vi "prep state ui.vi"(4 "Output Tag":refnum<vi>, 6 "Input Tag":refnum<vi>, 8 "error in":errorcluster, 10 "engine configuration in":refnum<class "engine configuration.lvclass">, 11 "user tag bus module configuration in":refnum<class "TEST CONFIGURATION.lvclass">) -> (0 "error out":errorcluster, 2 "engine configuration out":refnum<class "engine configuration.lvclass">)   [LabVIEW 2013, in "configuration tests.lvlib" / "TEST EDITOR.lvclass"]
uses:
  TEST EDITOR.lvclass
  module/configuration/TEST CONFIGURATION.lvclass
  <vilib>/NI/Module Execution Interface/Engine Configuration/engine configuration.lvclass
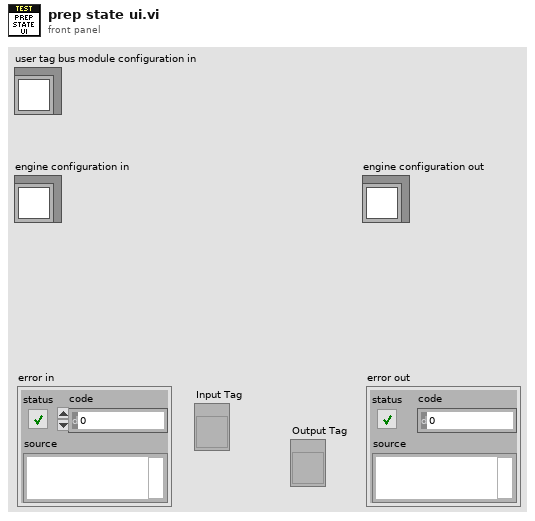
[diagram p1: front panel]
types:
  T1 = typedef "user tag bus module configuration.lvclass/state module configuration.ctl" = cluster{"fixed input":refnum<class "TBM channel.lvclass">, "fixed output":refnum<class "TBM channel.lvclass">, "initial state":u8}
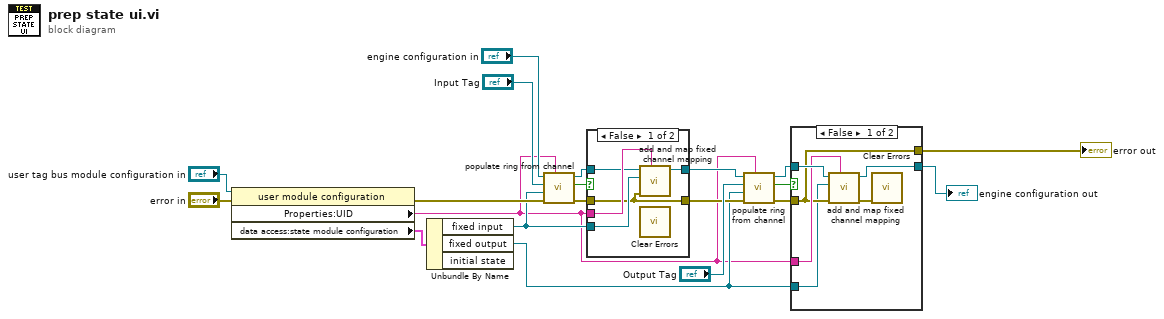
[diagram p0: block diagram]
diagram:
  n1 = property class="user module configuration"(reference="user tag bus module configuration in", error in="error in") -> (error out=w16:errorcluster, "Properties:UID"=w6:string, "data access:state module configuration"=w17:T1)  [unwired: 1 out]
  n2 = Unbundle By Name(w17) -> ("fixed input"=w10:refnum<class "TBM channel.lvclass">, "fixed output"=w7:refnum<class "TBM channel.lvclass">)  [unwired: 1 out]
  n3 = call "populate ring from channel.vi"("instance id"=w6, "error in"=w16, "channel"=w10, "ring"="Input Tag", "engine configuration in"="engine configuration in") -> ("error out"=w9:errorcluster, "mapped"=w13:bool, "engine configuration out"=w11:refnum<class "engine configuration.lvclass">)  [unwired: 4 in]
  n4 = case shown="False" w13 {
    tunnel: [w25 w27] -> w12
    tunnel: w11 -> [w22 w27]
    tunnel: w9 -> [w21 w26]
    tunnel: w10 -> [w24 _]
    tunnel: w6 -> [w23 _]
    tunnel: [w21 w26] -> w8
    frame False {
      n5 = call <vilib>:"add and map fixed channel mapping.vi"("module instance"=w23, "error in"=w21, "fixed channel"=w24, "engine configuration in"=w22) -> ("engine configuration out"=w25:refnum<class "engine configuration.lvclass">)  [unwired: 6 in, 1 out]
      n6 = call <vilib>:"Clear Errors.vi"() -> ()  [unwired: 7 in, 1 out]
    }
    frame True {
    }
  }
  n7 = call "populate ring from channel.vi"("instance id"=w6, "error in"=w8, "channel"=w7, "ring"="Output Tag", "engine configuration in"=w12) -> ("error out"=w3:errorcluster, "mapped"=w4:bool, "engine configuration out"=w5:refnum<class "engine configuration.lvclass">)  [unwired: 4 in]
  n8 = case shown="False" w4 {
    tunnel: [w28 w35] -> w2
    tunnel: w5 -> [w33 w35]
    tunnel: w3 -> [w31 w34]
    tunnel: w7 -> [w30 _]
    tunnel: w6 -> [w32 _]
    tunnel: [w31 w34] -> w1
    frame False {
      n9 = call <vilib>:"add and map fixed channel mapping.vi"("module instance"=w32, "error in"=w31, "fixed channel"=w30, "engine configuration in"=w33) -> ("error out"=w29:errorcluster, "engine configuration out"=w28:refnum<class "engine configuration.lvclass">)  [unwired: 6 in]
      n10 = call <vilib>:"Clear Errors.vi"("error in (no error)"=w29) -> ()  [unwired: 6 in, 1 out]
    }
    frame True {
    }
  }
  "error out" <- w1
  "engine configuration out" <- w2
